vi "Buffer_Extract from StartEnd and Duration.vi"(8 "Error":errorcluster, 9 "Duration(S)":dbl, 10 "From End(f)\nFrom Beginning(t)":bool, 11 "Buffer":T2) -> (0 "Error Out":errorcluster, 1 "End Index Out":i32, 2 "Start Index Out":i32, 3 "Waveform Out":T1)   [LabVIEW 2020]
doc: "Retrieves a subset of a waveform at a specified time or index. You must manually select the polymorphic instance you want to use."
uses:
  TypeDefs_Utility/Ref_DVR_Buffer.ctl
  Universal Controls/Waveform_Data.ctl
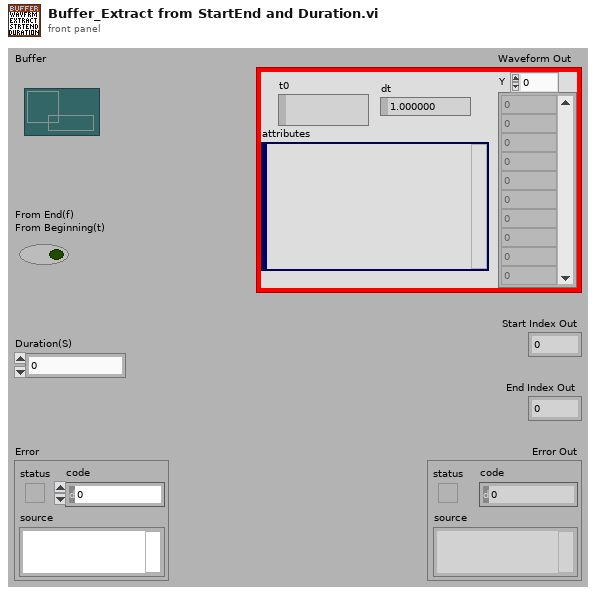
[diagram p1: front panel]
types:
  T1 = typedef "Waveform_Data.ctl" = waveform(dbl)
  T2 = typedef "Ref_DVR_Buffer.ctl" = refnum<data-value>
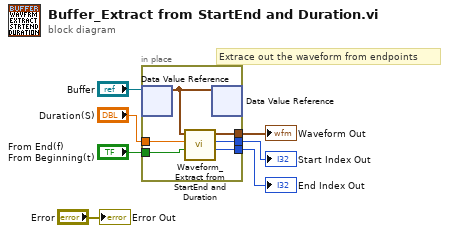
[diagram p0: block diagram]
diagram:
  # "Extrace out the waveform from endpoints"
  n1 = in-place {
    in-place-border: [w13] -> w6
    in-place-border: [w12] -> w5
    in-place-border: [w11] -> w4
    in-place-border: "From End(f)\nFrom Beginning(t)" -> [w10]
    in-place-border: "Duration(S)" -> [w9]
    n2 = in-place-dvr #1("Buffer") -> (w8:T1)  [unwired: 1 out]
    n3 = call "Waveform_Extract from StartEnd and Duration.vi"("From End(f)\nFrom Beginning(t)"=w10, "Duration(S)"=w9, "Raw Data Waveform"=w8) -> ("End Out"=w11:i32, "Start Out"=w12:i32, "Raw Data Waveform Out"=w13:T1)  [unwired: 6 in]
    n4 = in-place-dvr #1(w8) -> ()  [unwired: 2 out]
  }
  "Waveform Out" <- w6
  "Start Index Out" <- w5
  "End Index Out" <- w4
  "Error Out" <- "Error"
